vi "Set Last Step.vi"(8 "error in (no error)":errorcluster, 10 "Last Step":bool, 11 "Car Wash Controller in":refnum<class "Car Wash Controller.lvclass">) -> (0 "error out":errorcluster, 3 "Car Wash Controller out":refnum<class "Car Wash Controller.lvclass">)   [LabVIEW 2019, in "Car Wash Controller.lvlib" / "Car Wash Controller.lvclass"]
uses:
  Car Wash Controller.lvclass
  C:/Program Files (x86)/National Instruments/LabVIEW 2019/vi.lib/ActorFramework/Actor/Actor.lvclass
  <vilib>/ActorFramework/Actor/Actor.lvclass/Actor.ctl
  <vilib>/ActorFramework/Message Enqueuer/Message Enqueuer.lvclass/Message Enqueuer.ctl
  Car Wash Controller.lvclass/Car Wash Controller.ctl
  Sim Wash Display Console/Sim Wash Display Console Messages/Write Vehicle Out of Position Msg/Write Vehicle Out of Position Msg.lvclass/Write Vehicle Out of Position Msg.ctl
  Wash Steps.ctl
  Car Wash Controller Messages/Set Vehicle Position Msg/Set Vehicle Position Msg.lvclass/Set Vehicle Position Msg.ctl
  Sim Wash Display Console/Sim Wash Display Console Messages/Write Wash Step Indicator Msg/Write Wash Step Indicator Msg.lvclass/Write Wash Step Indicator Msg.ctl
  <vilib>/ActorFramework/Message Enqueuer/Init from Existing Queue.vi
  <vilib>/ActorFramework/Message Enqueuer/Enqueue.vi
  Sim Wash Display Console/Sim Wash Display Console Messages/Write Vehicle Out of Position Msg/Write Vehicle Out of Position Msg.lvclass
  C:/Program Files (x86)/National Instruments/LabVIEW 2019/vi.lib/ActorFramework/Message/Message.lvclass
  Car Wash Controller Messages/Set Vehicle Position Msg/Set Vehicle Position Msg.lvclass
  Sim Wash Display Console/Sim Wash Display Console Messages/Write Wash Step Indicator Msg/Write Wash Step Indicator Msg.lvclass
  <vilib>/ActorFramework/Message Priority Queue/Priority Enqueue.vi
  <vilib>/ActorFramework/Message Enqueuer/Message Enqueuer.lvclass
  <vilib>/ActorFramework/Actor/Actor.lvclass
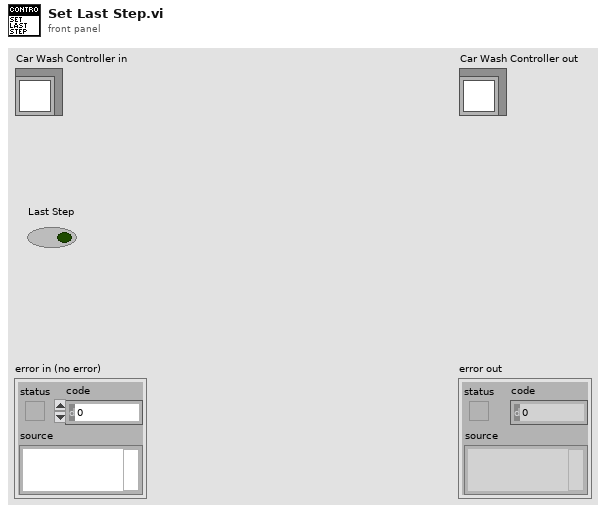
[diagram p1: front panel]
types:
  T1 = typedef "Car Wash Controller.lvlib/Car Wash Controller.lvclass/Wash Steps.ctl" = cluster{"Under Body Wash":bool, "Bug Remover":bool, "Pre-Soak":bool, "High Pressure Wash (Default)":bool, "Low Pressure Wax":bool, "Spot Free Rinse":bool, "Tire Shine Foam":bool, "Air Dry":bool}
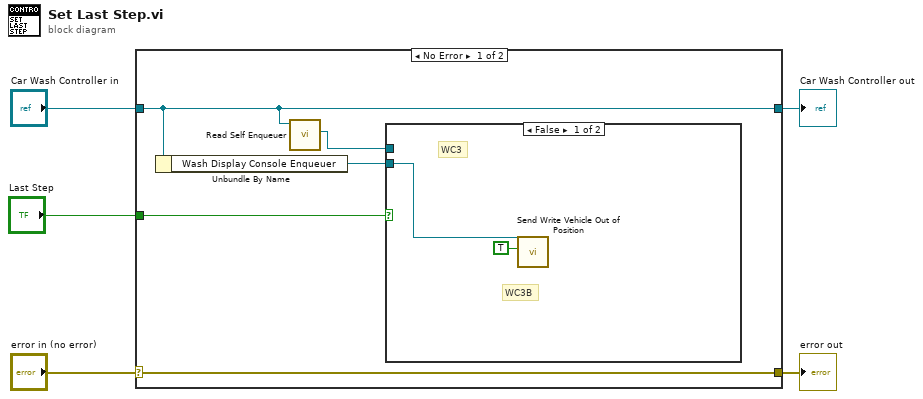
[diagram p0: block diagram]
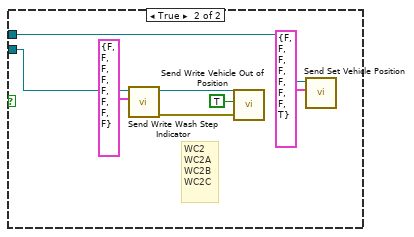
[diagram p2: hidden frame]
diagram:
  n1 = case shown="No Error" "error in (no error)" {
    selector: "error in (no error)" -> [w10 w21]
    tunnel: [w10 w21] -> w4
    tunnel: [w7 w20] -> w2
    tunnel: "Car Wash Controller in" -> [w7 w20]
    tunnel: "Last Step" -> [w9 _]
    frame No Error {
      n2 = Unbundle By Name(w7) -> ("Wash Display Console Enqueuer"=w8:refnum<class "Message Enqueuer.lvclass">)
      n3 = call <vilib>:"Read Self Enqueuer.vi"("Actor"=w7) -> ("Self Enqueuer"=w6:refnum<class "Message Enqueuer.lvclass">)  [unwired: 10 in]
      n4 = case shown="False" w9 {
        tunnel: w8 -> [w11 w19]
        tunnel: w6 -> [_ w14]
        frame False {
          # "WC3"
          # "WC3B"
          n5 = call "Send Write Vehicle Out of Position.vi"("Vehicle Out of Position"=TRUE, "Message Enqueuer"=w11) -> ()  [unwired: 8 in, 2 out]
        }
        frame True {
          # "WC2\nWC2A\nWC2B\nWC2C"
          n6 = call "Send Write Wash Step Indicator.vi"("Wash Steps"=T1 {"Under Body Wash"=FALSE, "Bug Remover"=FALSE, "Pre-Soak"=FALSE, "High Pressure Wash (Default)"=FALSE, "Low Pressure Wax"=FALSE, "Spot Free Rinse"=FALSE, "Tire Shine Foam"=FALSE, "Air Dry"=FALSE}, "Message Enqueuer"=w19) -> ("error out"=w16:errorcluster, "Message Enqueuer out"=w17:refnum<class "Message Enqueuer.lvclass">)  [unwired: 8 in]
          n7 = call "Send Write Vehicle Out of Position.vi"("error in (no error)"=w16, "Vehicle Out of Position"=TRUE, "Message Enqueuer"=w17) -> ()  [unwired: 7 in, 2 out]
          n8 = call "Send Set Vehicle Position.vi"("Wash Steps"=T1 {"Under Body Wash"=FALSE, "Bug Remover"=FALSE, "Pre-Soak"=FALSE, "High Pressure Wash (Default)"=FALSE, "Low Pressure Wax"=FALSE, "Spot Free Rinse"=FALSE, "Tire Shine Foam"=FALSE, "Air Dry"=TRUE}, "Message Enqueuer"=w14) -> ()  [unwired: 8 in, 2 out]
        }
      }
    }
    frame Error {
    }
  }
  "error out" <- w4
  "Car Wash Controller out" <- w2
